vi "img test3.vi"() -> ()   [LabVIEW 2009]
uses:
  <vilib>/vision/NI_Vision_Development_Module.lvlib
panel:
  out "x+y":i32
  in  "Empty frame":u32
  in  "Range 2":cluster{"Lower value":sgl, "Upper value":sgl}={"Lower value"=0.0, "Upper value"=100.0} {"Upper value" format="%.2f"; "Lower value" format="%.2f"}
  out "Image Pixels (U8)":u8[][](array[numeric])
  in  "Number of Erosion":i32=1
  out "Image 6":T1(plugin-control)
  in  "Number of iterations (1) 4":i32=8
  in  "Structuring Element 4":i32[][](array[numeric])=[[1, 1, 1, 1, 1], [0, 0, 1, 0, 0], [0, 0, 1, 0, 0], [0, 0, 1, 0, 0], [1, 1, 1, 1, 1]]
  in  "Operation 4":T2(ring)=enum."Erode"
  out "Image 5":T1(plugin-control)
  in  "Number of iterations (1) 3":i32=3
  in  "Structuring Element 3":i32[][](array[numeric])=[[1, 0, 1, 0, 1], [0, 1, 1, 1, 0], [0, 0, 1, 0, 0], [0, 1, 1, 1, 0], [1, 0, 1, 0, 1]]
  in  "Operation 3":T2(ring)=enum."Dilate"
  out "Image 4":T1(plugin-control)
  in  "Number of iterations (1) 2":i32=3
  in  "Structuring Element 2":i32[][](array[numeric])=[[0, 0, 1, 0, 0], [0, 0, 1, 0, 0], [0, 0, 1, 0, 0], [0, 0, 1, 0, 0], [0, 0, 1, 0, 0]]
  in  "Operation 2":T2(ring)=enum."Dilate"
  in  "Operation 1":T2(ring)=enum."Dilate"
  in  "Structuring Element":i32[][](array[numeric])=[[1, 1, 1, 1, 1], [1, 0, 0, 0, 1], [1, 0, 0, 0, 1], [1, 0, 0, 0, 1], [1, 1, 1, 1, 1]]
  in  "Number of iterations (1)":i32=1
  out "Image 3":T1(plugin-control)
  out "Image":T1(plugin-control)
  in  "Range":cluster{"Lower value":sgl, "Upper value":sgl}={"Lower value"=0.0, "Upper value"=100.0} {"Upper value" format="%.2f"; "Lower value" format="%.2f"}
  in  "stop":bool
  out "Image 2":T1(plugin-control)
  in  "startign rame":i32
  in  "AVI Path":path=path "C:/Users/Kokum Weeratunga/Desktop/img processing/ChongWei vs LinDan (japan open 2010).avi"
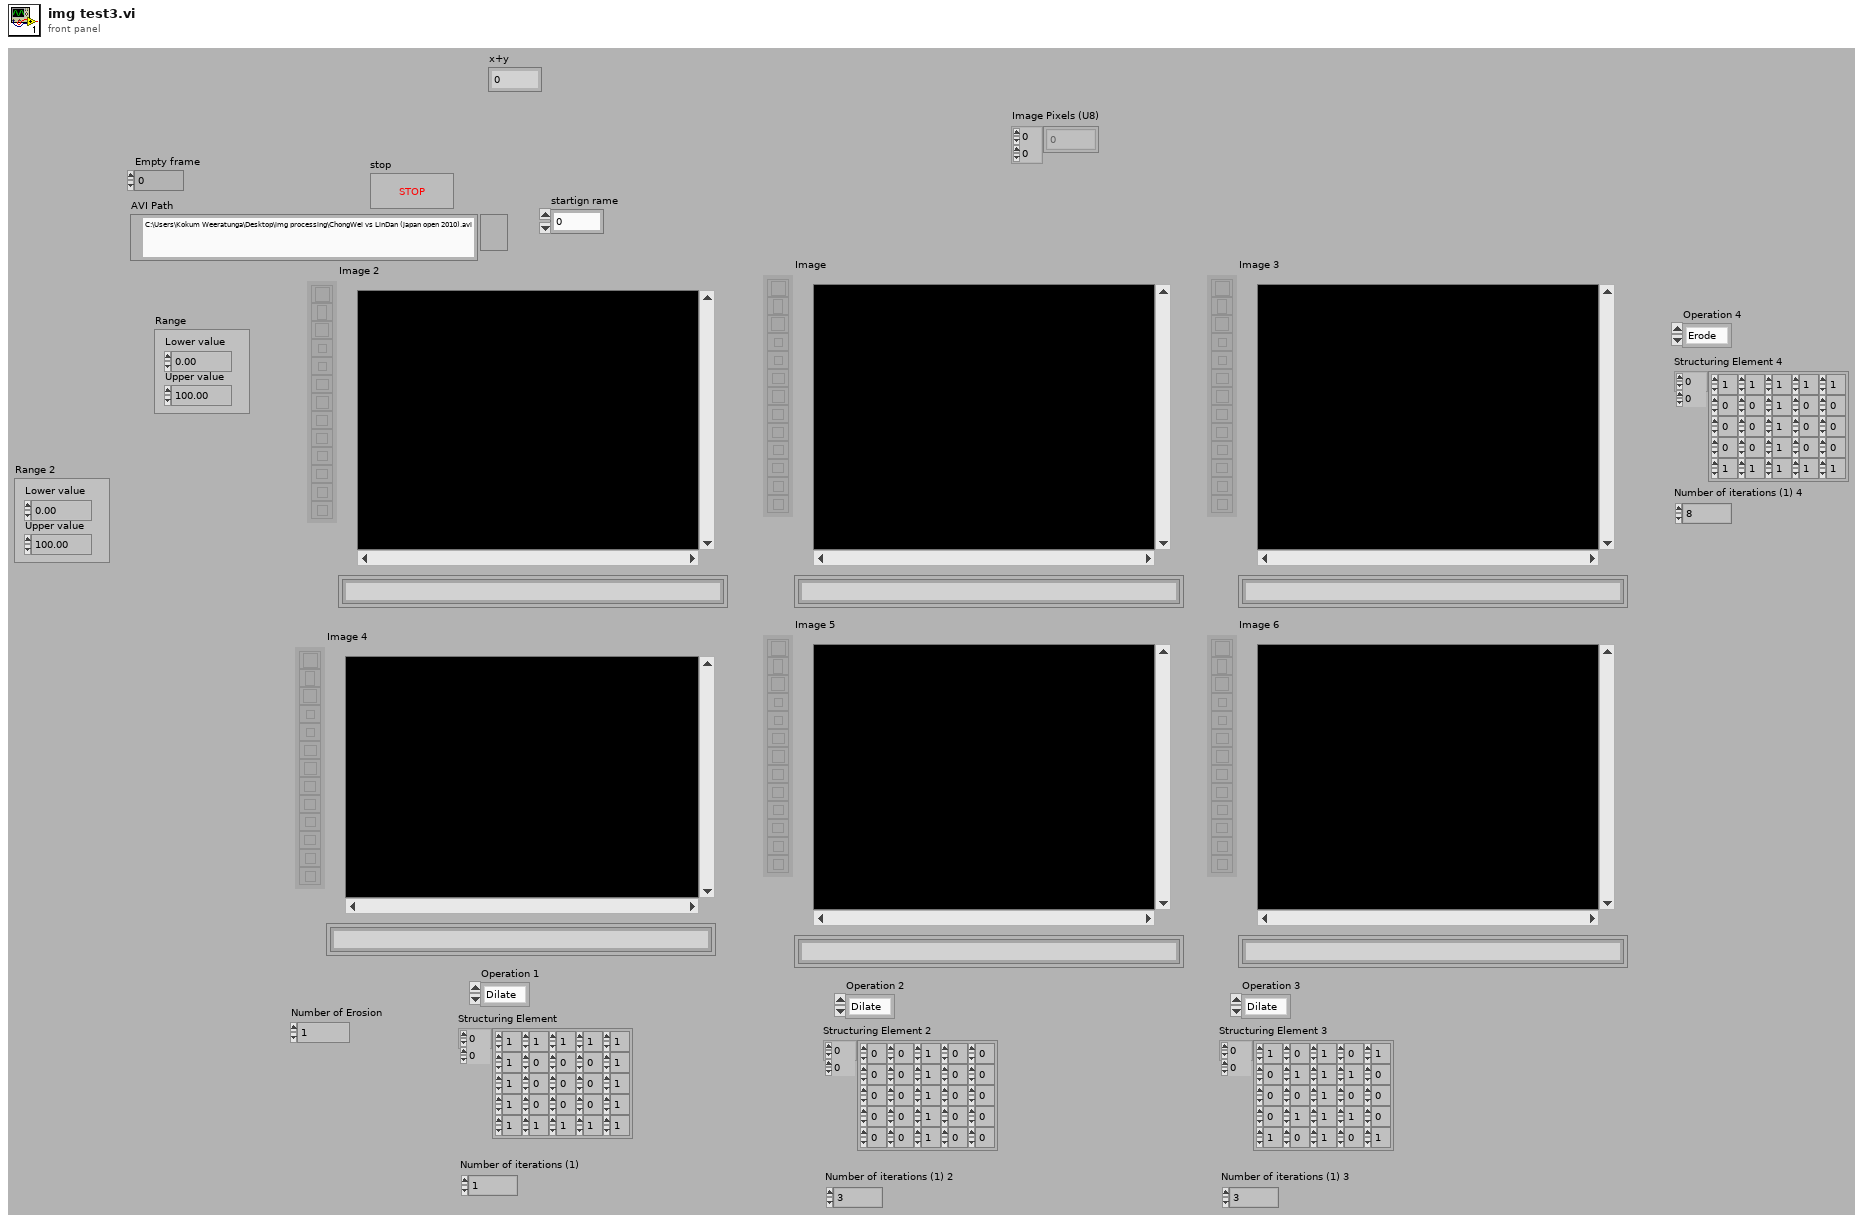
[diagram p1: front panel]
types:
  T1 = typedef "IMAQ Image.ctl" = refnum<image>
  T2 = enum32{"AutoM", "Close", "Dilate", "Erode", "Gradient", "Gradient in", "Gradient out", "HitMiss", "Open", "PClose", "POpen", "Thick", "Thin"}
  T3 = typedef "Image Type" = u32
  T4 = typedef "AviRefnum.ctl" = refnum<k1>
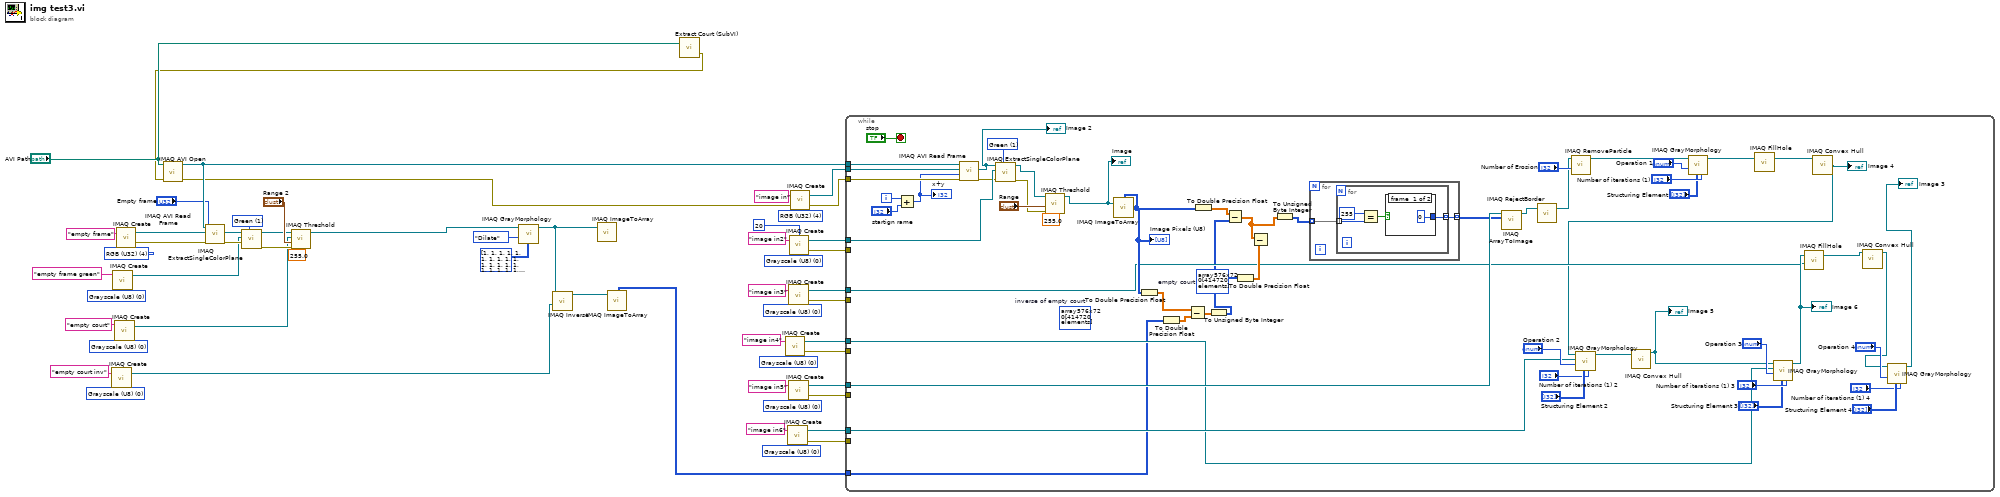
[diagram p0: block diagram]
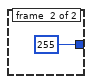
[diagram p2: hidden frame]
diagram:
  w13 = T3 0 items=["Grayscale (U8)", "Grayscale (I16)", "Grayscale (SGL)", "Complex (CSG)", "RGB (U32)", "HSL (U32)", "RGB (U64)", "Grayscale (U16)"] ("Image Type")
  w21 = T3 0 items=["Grayscale (U8)", "Grayscale (I16)", "Grayscale (SGL)", "Complex (CSG)", "RGB (U32)", "HSL (U32)", "RGB (U64)", "Grayscale (U16)"] ("Image Type")
  w20 = T3 0 items=["Grayscale (U8)", "Grayscale (I16)", "Grayscale (SGL)", "Complex (CSG)", "RGB (U32)", "HSL (U32)", "RGB (U64)", "Grayscale (U16)"] ("Image Type")
  w8 = T3 4 items=["Grayscale (U8)", "Grayscale (I16)", "Grayscale (SGL)", "Complex (CSG)", "RGB (U32)", "HSL (U32)", "RGB (U64)", "Grayscale (U16)"] ("Image Type")
  w33 = 1 items=["Red", "Green", "Blue", "Hue", "Saturation", "Luminance", "Value", "Intensity"] ("Color Plane")
  w36 = T3 0 items=["Grayscale (U8)", "Grayscale (I16)", "Grayscale (SGL)", "Complex (CSG)", "RGB (U32)", "HSL (U32)", "RGB (U64)", "Grayscale (U16)"] ("Image Type")
  w47 = T3 0 items=["Grayscale (U8)", "Grayscale (I16)", "Grayscale (SGL)", "Complex (CSG)", "RGB (U32)", "HSL (U32)", "RGB (U64)", "Grayscale (U16)"] ("Image Type")
  w45 = T3 0 items=["Grayscale (U8)", "Grayscale (I16)", "Grayscale (SGL)", "Complex (CSG)", "RGB (U32)", "HSL (U32)", "RGB (U64)", "Grayscale (U16)"] ("Image Type")
  w49 = T3 0 items=["Grayscale (U8)", "Grayscale (I16)", "Grayscale (SGL)", "Complex (CSG)", "RGB (U32)", "HSL (U32)", "RGB (U64)", "Grayscale (U16)"] ("Image Type")
  w51 = T3 0 items=["Grayscale (U8)", "Grayscale (I16)", "Grayscale (SGL)", "Complex (CSG)", "RGB (U32)", "HSL (U32)", "RGB (U64)", "Grayscale (U16)"] ("Image Type")
  w53 = T3 4 items=["Grayscale (U8)", "Grayscale (I16)", "Grayscale (SGL)", "Complex (CSG)", "RGB (U32)", "HSL (U32)", "RGB (U64)", "Grayscale (U16)"] ("Image Type")
  n1 = call "IMAQ Create"("Image Name"="empty court inv", "Image Type"=w21) -> ("New Image"=w23:T1)  [unwired: 3 in, 1 out]
  n2 = call "IMAQ Create"("Image Name"="empty frame green", "Image Type"=w13) -> ("New Image"=w12:T1)  [unwired: 3 in, 1 out]
  n3 = call "IMAQ Create"("Image Name"="empty court", "Image Type"=w20) -> ("New Image"=w11:T1)  [unwired: 3 in, 1 out]
  n4 = call "IMAQ Create"("Image Name"="empty frame", "Image Type"=w8) -> ("New Image"=w25:T1, "error out"=w24:errorcluster)  [unwired: 3 in]
  n5 = call "Extract Court (SubVI).vi"("AVI Path"="AVI Path") -> ("error out"=w3:errorcluster)  [unwired: 1 in, 1 out]
  n6 = call "IMAQ AVI Open"("error in (no error)"=w3, "AVI Path"="AVI Path") -> ("error out"=w27:errorcluster, "Avi Refnum"=w28:T4)  [unwired: 8 in]
  n7 = call "IMAQ AVI Read Frame"("error in (no error)"=w24, "Frame Number"="Empty frame", "Image"=w25, "Avi Refnum"=w28) -> ("error out"=w31:errorcluster, "Image Out"=w10:T1)  [unwired: 4 in, 2 out]
  n8 = call "IMAQ ExtractSingleColorPlane"("Color Plane"=w33, "error in (no error)"=w31, "Image Dst"=w12, "Image Src"=w10) -> ("error out"=w32:errorcluster, "Image Dst Out"=w9:T1)  [unwired: 6 in]
  n9 = call "IMAQ Threshold"("Replace Value"=sgl 255.0, "error in (no error)"=w32, "Range"="Range 2", "Image Dst"=w11, "Image Src"=w9) -> ("Image Dst Out"=w1:T1)  [unwired: 5 in, 1 out]
  n10 = call "IMAQ GrayMorphology"("Structuring Element"=i32[][] [[1, 1, 1, 1, 1], [1, 1, 1, 1, 1], [1, 1, 1, 1, 1], [1, 1, 1, 1, 1], [1, 1, 1, 1, 1]], "Operation"=T2."Dilate" ("Operation 1"), "Image Src"=w1) -> ("Image Dst Out"=w6:T1)  [unwired: 7 in, 1 out]
  n11 = call "IMAQ Inverse"("Image Dst"=w23, "Image Src"=w6) -> ("Image Dst Out"=w15:T1)  [unwired: 8 in, 1 out]
  n12 = call "IMAQ ImageToArray"("Image"=w6) -> ()  [unwired: 3 in, 5 out]
  n13 = call "IMAQ ImageToArray"("Image"=w15) -> ("Image Pixels (U8)"=w5:u8[][])  [unwired: 3 in, 4 out]
  n14 = call "IMAQ Create"("Image Name"="image in4", "Image Type"=w47) -> ("New Image"=w41:T1, "error out"=w40:errorcluster)  [unwired: 3 in]
  n15 = call "IMAQ Create"("Image Name"="image in6", "Image Type"=w36) -> ("New Image"=w35:T1, "error out"=w34:errorcluster)  [unwired: 3 in]
  n16 = call "IMAQ Create"("Image Name"="image in3", "Image Type"=w45) -> ("New Image"=w43:T1, "error out"=w42:errorcluster)  [unwired: 3 in]
  n17 = call "IMAQ Create"("Image Name"="image in5", "Image Type"=w49) -> ("New Image"=w39:T1, "error out"=w38:errorcluster)  [unwired: 3 in]
  n18 = call "IMAQ Create"("Border Size"=20, "Image Name"="image in2", "Image Type"=w51) -> ("New Image"=w2:T1, "error out"=w50:errorcluster)  [unwired: 2 in]
  n19 = call "IMAQ Create"("Image Name"="image in", "Image Type"=w53, "error in (no error)"=w27) -> ("New Image"=w54:T1, "error out"=w55:errorcluster)  [unwired: 2 in]
  n20 = while {
    tunnel: w55 -> [w113]
    tunnel: w54 -> [w112]
    tunnel: w28 -> [w108]
    tunnel: w2 -> [w102]
    tunnel: w50 -> [_]
    tunnel: w43 -> [w68]
    tunnel: w42 -> [_]
    tunnel: w41 -> [w76]
    tunnel: w40 -> [_]
    tunnel: w39 -> [w103]
    tunnel: w38 -> [_]
    tunnel: w35 -> [w80]
    tunnel: w34 -> [_]
    tunnel: w5 -> [w57]
    i -> [w107]
    stop <- "stop" stop-if-true
    (unwired) u8[][] array576x720[414720 elements]  # inverse of empty court
    w95 = u8[][] array576x720[414720 elements]  # empty court
    w99 = 1 items=["Red", "Green", "Blue", "Hue", "Saturation", "Luminance", "Value", "Intensity"] ("Color Plane")
    n21 = Add(x=w107, y="startign rame") -> (x+y=w105:i32)
    "x+y" <- w105
    n22 = call "IMAQ AVI Read Frame"("error in (no error)"=w113, "Frame Number"=w105, "Image"=w112, "Avi Refnum"=w108) -> ("error out"=w101:errorcluster, "Image Out"=w87:T1)  [unwired: 4 in, 2 out]
    "Image 2" <- w87
    n23 = call "IMAQ ExtractSingleColorPlane"("Color Plane"=w99, "error in (no error)"=w101, "Image Dst"=w102, "Image Src"=w87) -> ("error out"=w100:errorcluster, "Image Dst Out"=w92:T1)  [unwired: 6 in]
    n24 = call "IMAQ Threshold"("Replace Value"=sgl 255.0, "error in (no error)"=w100, "Range"="Range", "Image Src"=w92) -> ("Image Dst Out"=w58:T1)  [unwired: 6 in, 1 out]
    "Image" <- w58
    n25 = call "IMAQ ImageToArray"("Image"=w58) -> ("Image Pixels (U8)"=w86:u8[][])  [unwired: 3 in, 4 out]
    "Image Pixels (U8)" <- w86
    n26 = To Double Precision Float(number=w86) -> (double precision float=w89:dbl[][])
    n27 = To Double Precision Float(number=w57) -> (double precision float=w90:dbl[][])
    n28 = Subtract(x=w89, y=w90) -> (x-y=w88:dbl[][])
    n29 = To Double Precision Float(number=w86) -> (double precision float=w104:dbl[][])
    n30 = To Unsigned Byte Integer(number=w88) -> (unsigned 8bit integer=w67:u8[][])
    n31 = Subtract(x=w104, y=w67) -> (x-y=w84:dbl[][])
    n32 = To Double Precision Float(number=w95) -> (double precision float=w85:dbl[][])
    n33 = Subtract(x=w84, y=w85) -> ()  [unwired: 1 out]
    n34 = To Unsigned Byte Integer(number=w84) -> (unsigned 8bit integer=w94:u8[][])
    n35 = for {
      tunnel: w94 -> [w115] mode=indexing
      tunnel: [w114] -> w93 mode=indexing
      n36 = for {
        tunnel: w115 -> [w119] mode=indexing
        tunnel: [w116] -> w114 mode=indexing
        n37 = Equal?(x=u8 255, y=w119) -> (x = y?=w117:bool)
        n38 = case shown="False" w117 {
          tunnel: [u8 0 ("x") u8 255 ("x")] -> w116
          frame #0 {
          }
          frame #1 {
          }
        }
      }
    }
    n39 = call "IMAQ ArrayToImage"("Image Pixels (U8)"=w93, "Image"=w103) -> ("Image Out"=w91:T1)  [unwired: 8 in, 1 out]
    n40 = call "IMAQ RejectBorder"("Image Src"=w91) -> ("Image Dst Out"=w63:T1)  [unwired: 5 in, 1 out]
    n41 = call "IMAQ RemoveParticle"("Number of Erosion"="Number of Erosion", "Image Src"=w63) -> ("Image Dst Out"=w62:T1)  [unwired: 8 in, 1 out]
    n42 = call "IMAQ GrayMorphology"("Number of iterations (1)"="Number of iterations (1)", "Structuring Element"="Structuring Element", "Operation"="Operation 1", "Image Src"=w62) -> ("Image Dst Out"=w61:T1)  [unwired: 6 in, 1 out]
    n43 = call "IMAQ FillHole"("Image Src"=w61) -> ("Image Dst Out"=w65:T1)  [unwired: 5 in, 1 out]
    n44 = call "IMAQ Convex Hull"("Image Src"=w65) -> ("Image Dst Out"=w64:T1)  [unwired: 9 in, 1 out]
    "Image 4" <- w64
    n45 = call "IMAQ GrayMorphology"("Number of iterations (1)"="Number of iterations (1) 2", "Structuring Element"="Structuring Element 2", "Operation"="Operation 2", "Image Dst"=w80, "Image Src"=w64) -> ("Image Dst Out"=w60:T1)  [unwired: 5 in, 1 out]
    n46 = call "IMAQ Convex Hull"("Image Src"=w60) -> ("Image Dst Out"=w59:T1)  [unwired: 9 in, 1 out]
    "Image 5" <- w59
    n47 = call "IMAQ GrayMorphology"("Number of iterations (1)"="Number of iterations (1) 3", "Structuring Element"="Structuring Element 3", "Operation"="Operation 3", "Image Dst"=w76, "Image Src"=w59) -> ("Image Dst Out"=w69:T1)  [unwired: 5 in, 1 out]
    "Image 6" <- w69
    n48 = call "IMAQ FillHole"("Image Dst"=w68, "Image Src"=w69) -> ("Image Dst Out"=w75:T1)  [unwired: 4 in, 1 out]
    n49 = call "IMAQ Convex Hull"("Image Src"=w75) -> ("Image Dst Out"=w70:T1)  [unwired: 9 in, 1 out]
    n50 = call "IMAQ GrayMorphology"("Number of iterations (1)"="Number of iterations (1) 4", "Structuring Element"="Structuring Element 4", "Operation"="Operation 4", "Image Src"=w70) -> ("Image Dst Out"=→"Image 3":T1)  [unwired: 6 in, 1 out]
  }
